vi "Q Vision_2017 Object Distance Cal_Pixel Sum.vi"(11 "Pixel Sum":i32) -> (3 "Distance (ft)":dbl)   [LabVIEW 2016]
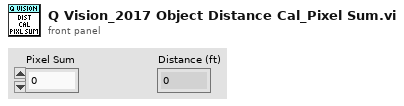
[diagram p1: front panel]
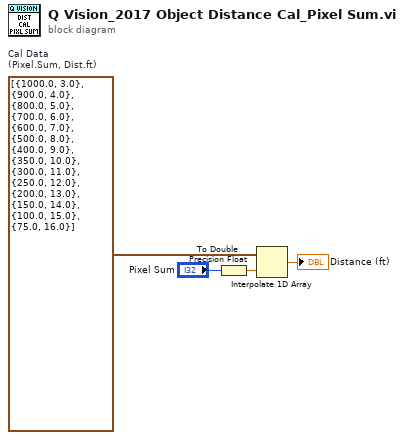
[diagram p0: block diagram]
diagram:
  w4 = cluster{dbl, dbl}[] [{1000.0, 3.0}, {900.0, 4.0}, {800.0, 5.0}, {700.0, 6.0}, {600.0, 7.0}, {500.0, 8.0}, {400.0, 9.0}, {350.0, 10.0}, {300.0, 11.0}, {250.0, 12.0}, {200.0, 13.0}, {150.0, 14.0}, {100.0, 15.0}, {75.0, 16.0}]  # Cal Data (Pixel.Sum, Dist.ft)
  n1 = To Double Precision Float(number="Pixel Sum") -> (double precision float=w2:dbl)
  n2 = Interpolate 1D Array(1:w2, 2:w4) -> (0:→"Distance (ft)":dbl)
